vi "OptoSpike.vi"(8 "Threshold (mV)":dbl, 9 "Parameters for Optic stimulation":T1, 10 "Path of ABF file":path=path "C:/Users/KimYG/Documents/카카오톡 받은 파일/JJ_Ask for/PV_KO_Patch+other_10Hz_5ms.abf", 11 "OptoSpike Cluster IN":T2) -> (3 "OptoSpike Cluster OUT":T2)   [LabVIEW 2017]
uses:
  OptoSpike Cluster.ctl
  Parameters for Optic Stimulation.ctl
  <vilib>/addons/Wavelet Analysis/application.llb/WA Multiscale Peak Detection (Array).vi
  <vilib>/addons/_Advanced Signal Processing/NI_AdvSigProcWA.lvlib
panel:
  out "Epoch":sgl[][](graph)
  out "InterSpike Interval (sec)":string="1\t10\t100\n2\t11\t110\n3\t12\t120\n4\t13\t130\n5\t14\t140\n6\t15\t150\n7\t16\t160\n8\t17\t170\n9\t18\t180\n"
  out "Summary Table":string[][](table)
  out "Raster plot":cluster{"location":dbl[], i32[]}[](graph)
  out "File Paramters":T3
  out "Whole Trace":sgl[][](graph)
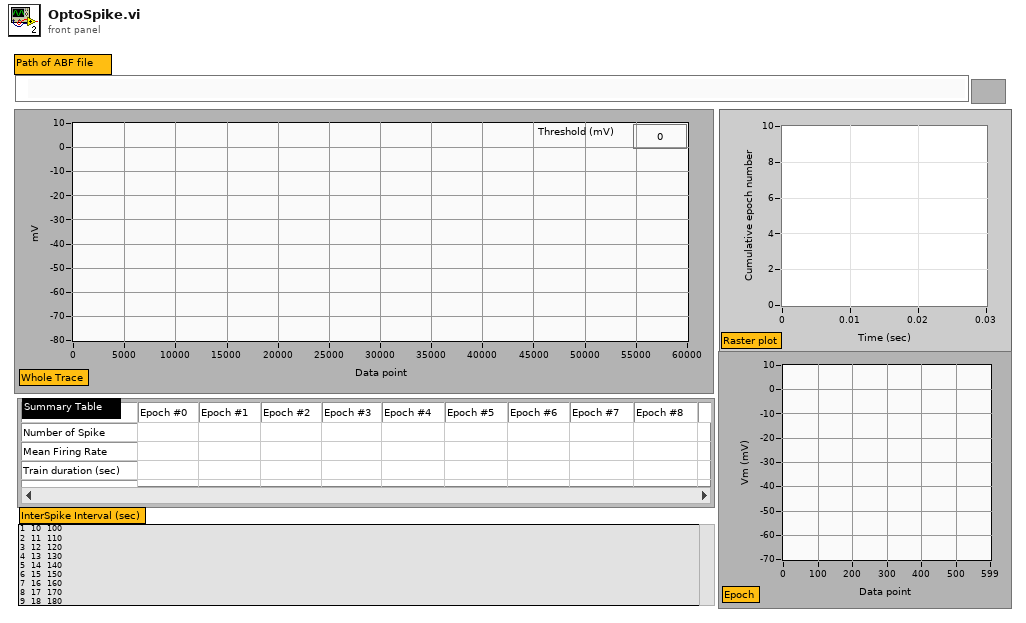
[diagram p1: front panel]
types:
  T1 = typedef "Parameters for Optic Stimulation.ctl" = cluster{"Begin (sec)":string, "Frequency (Hz)":string, "Epoch":string, "Time window (ms)":string}
  T2 = typedef "OptoSpike Cluster.ctl" = cluster{"File Paramters":cluster{"File Path":path, "Cell ID":string, "File Name":string, "Total Length":i32, "Trial Length (ms)":dbl, "Sweep Number":dbl, "Sampling rate":dbl}, "Raster Plot":cluster{"location":dbl[], "Sweep":i32[]}[], "Summary Table":string[][], "Pooled ISI":dbl[]}
  T3 = cluster{"File Path":path, "Cell ID":string, "File Name":string, "Total Length":i32, "Trial Length (ms)":dbl, "Sweep Number":dbl, "Sampling rate":dbl}
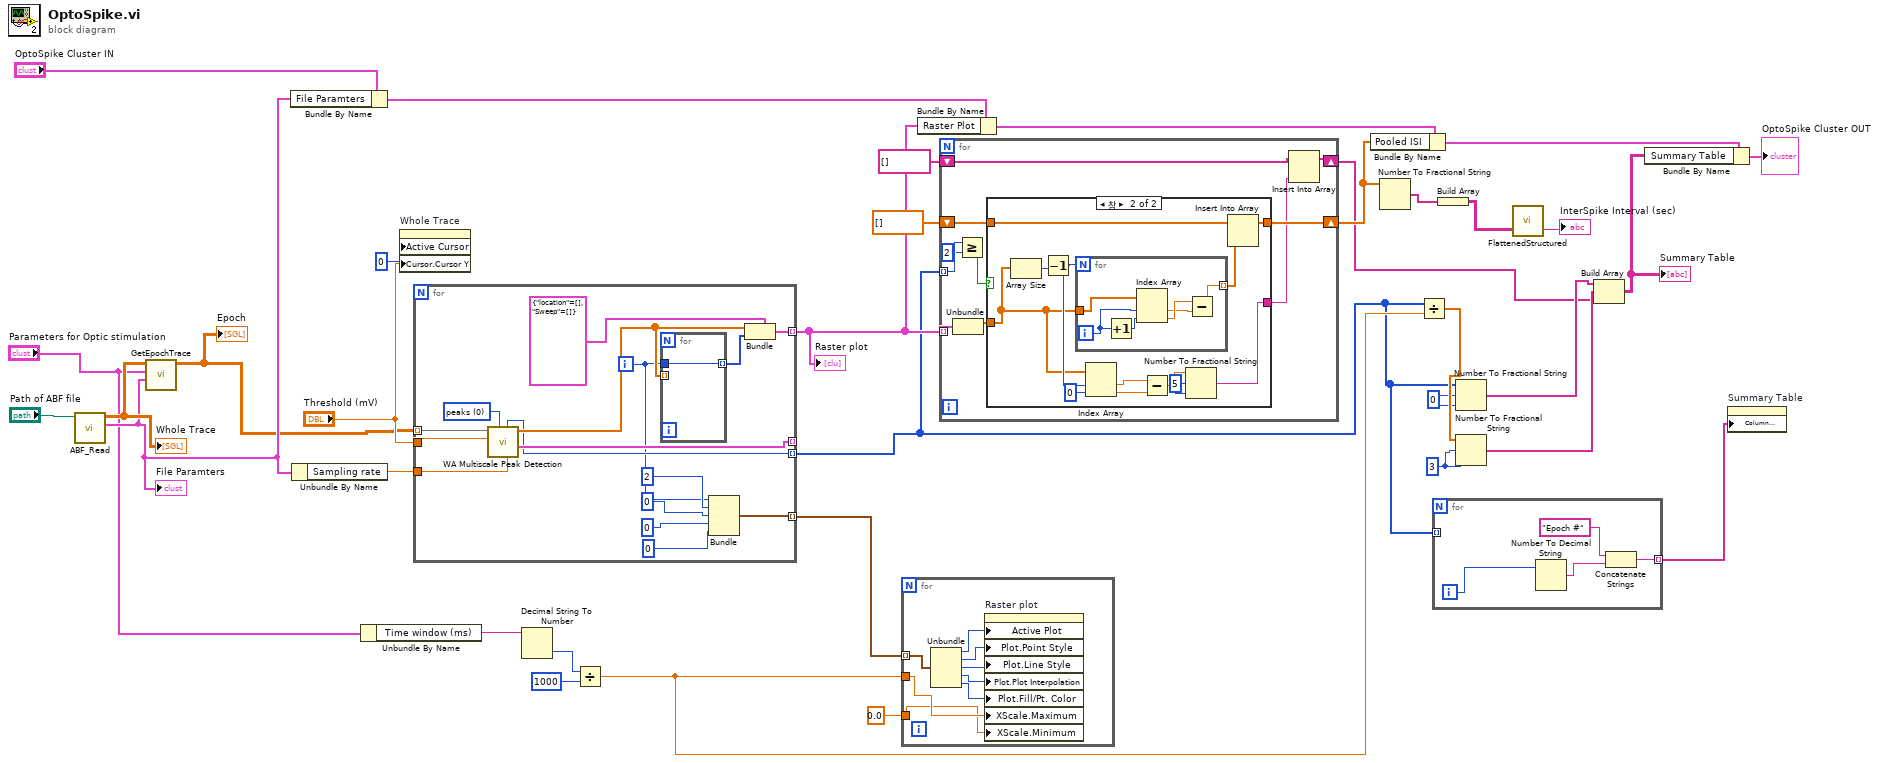
[diagram p0: block diagram]
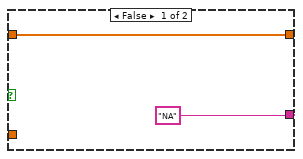
[diagram p2: hidden frame]
diagram:
  w7 = i16 3 ("폭(-)")
  w8 = i16 0 ("폭(-)")
  n1 = call "ABF_Read.vi"("Path of ABF file"="Path of ABF file") -> ("File Paramters"=w25:T3, "Whole Trace"=w26:sgl[][])  [unwired: 4 in, 1 out]
  "Whole Trace" <- w26
  "File Paramters" <- w25
  n2 = call "GetEpochTrace.vi"("File Paramters"=w25, "Parameters for Optic stimulation"="Parameters for Optic stimulation", "Whole Trace"=w26) -> ("Epoch"=w3:sgl[][])  [unwired: 4 in]
  "Epoch" <- w3
  n3 = Bundle By Name(cluster="OptoSpike Cluster IN", "File Paramters"=w25) -> (w32:T2)
  n4 = Unbundle By Name(w25) -> ("Sampling rate"=w20:dbl)
  n5 = Unbundle By Name("Parameters for Optic stimulation") -> ("Time window (ms)"=w22:string)
  n6 = property on="Whole Trace" class="WFGraph (엄격한)"("Active Cursor"=u32 0 ("활성 커서"), "Cursor.Cursor Y"="Threshold (mV)") -> ()  [unwired: 2 in, 2 out]
  n7 = for {
    tunnel: w3 -> [w51] mode=indexing
    tunnel: "Threshold (mV)" -> [w50]
    tunnel: [w48] -> _ mode=indexing
    tunnel: w20 -> [w47]
    tunnel: [w44] -> w27 mode=indexing
    tunnel: [w43] -> w5 mode=indexing
    tunnel: [w36] -> w24 mode=indexing
    i -> [w37]
    w49 = u16 0 items=["peaks", "valleys"] ("peaks/valleys")
    n8 = call-poly <vilib>:"WA Multiscale Peak Detection.vi"("sampling rate"=w47, "peaks/valleys"=w49, "threshold"=w50, "signal"=w51) -> ("peak plot"=w48:cluster{"Ramp Pattern":dbl[], "X":dbl[]}[], "location"=w46:dbl[], "number of peaks"=w43:i32)  [unwired: 3 in, 2 out]
    n9 = for {
      tunnel: w46 -> [_] mode=indexing
      tunnel: w37 -> [w52]
      tunnel: [w52] -> w45 mode=indexing
    }
    n10 = Bundle(w37, u8 2, u8 0, u8 0, u32 0) -> (w36:cluster{i32, u8, u8, u8, u32})  [unwired: 1 in]
    n11 = Bundle(cluster=cluster{"location":dbl[], "Sweep":i32[]} {"location"=[], "Sweep"=[]} ("클러스터"), "location"=w46, "Sweep"=w45) -> (w44:cluster{"location":dbl[], "Sweep":i32[]})
  }
  "Raster plot" <- w27
  n12 = Decimal String To Number(string=w22) -> (number=w21:i32)  [unwired: 2 in, 1 out]
  n13 = Divide(x=w21, y=1000) -> (x/y=w17:dbl)
  n14 = for {
    tunnel: w24 -> [w60] mode=indexing
    tunnel: w17 -> [w54]
    tunnel: 0.0 -> [w53]
    n15 = Unbundle(w60) -> (w59:i32, w58:u8, w57:u8, w56:u8, w55:u32)
    n16 = property on="Raster plot" class="XYGraph (엄격한)"("Active Plot"=w59, "Plot.Point Style"=w58, "Plot.Line Style"=w57, "Plot.Plot Interpolation"=w56, "Plot.Fill/Pt. Color"=w55, "XScale.Maximum"=w54, "XScale.Minimum"=w53) -> ()  [unwired: 2 in, 2 out]
  }
  n17 = Bundle By Name(cluster=w32, "Raster Plot"=w27) -> (w31:T2)
  n18 = for {
    tunnel: w27 -> [w70] mode=indexing
    shift-right: [w65] -> w15
    shift-left: dbl[] [] -> [w64]
    tunnel: w5 -> [w68] mode=indexing
    shift-right: [w62] -> w2
    shift-left: string[] [] -> [w61]
    n19 = Unbundle(w70) -> ("location"=w69:dbl[])  [unwired: 1 out]
    n20 = Greater Or Equal?(x=w68, y=2) -> (x >= y?=w66:bool)
    n21 = case shown="참" w66 {
      tunnel: w69 -> [_ w78]
      tunnel: w64 -> [w72 w81]
      tunnel: [w72 w82] -> w65
      tunnel: ["NA" w74] -> w63
      frame False {
      }
      frame True {
        w73 = i16 5 ("폭(-)")
        n22 = Array Size(array=w78) -> (size(s)=w84:i32)
        n23 = Decrement(x=w84) -> (x-1=w80:i32)
        n24 = for {
          N: w80 -> [_]
          tunnel: w78 -> [w90]
          tunnel: [w85] -> w83 mode=indexing
          i -> [w89]
          n25 = Increment(x=w89) -> (x+1=w88:i32)
          n26 = Index Array(array=w90, index #1=w89, index #2=w88) -> (element #1=w86:dbl, element #2=w87:dbl)
          n27 = Subtract(x=w87, y=w86) -> (x-y=w85:dbl)
        }
        n28 = Index Array(array=w78, index #1=w80, index #2=0 ("인덱스")) -> (element #1=w77:dbl, element #2=w76:dbl)
        n29 = Subtract(x=w77, y=w76) -> (x-y=w75:dbl)
        n30 = Number To Fractional String(number=w75, width (-)=w73, precision (6)=w73) -> (F-format string=w74:string)  [unwired: 1 in]
        n31 = Insert Into Array(array=w81, new element=w83) -> (w82:dbl[])  [unwired: 1 in]
      }
    }
    n32 = Insert Into Array(array=w61, new element=w63) -> (w62:string[])  [unwired: 1 in]
  }
  n33 = Bundle By Name(cluster=w31, "Pooled ISI"=w15) -> (w30:T2)
  n34 = Number To Fractional String(number=w15) -> (F-format string=w14:string[])  [unwired: 3 in]
  n35 = Divide(x=w5, y=w17) -> (x/y=w10:dbl[])
  n36 = for {
    tunnel: w5 -> [_] mode=indexing
    tunnel: [w91] -> w4 mode=indexing
    i -> [w94]
    n37 = Number To Decimal String(number=w94) -> (decimal integer string=w92:string)  [unwired: 1 in]
    n38 = Concatenate Strings("Epoch #", w92) -> (w91:string)
  }
  n39 = Build Array(w14) -> (w13:string[][])
  n40 = Number To Fractional String(number=w5, width (-)=w8, precision (6)=w8) -> (F-format string=w11:string[])  [unwired: 1 in]
  n41 = Number To Fractional String(number=w10, width (-)=w7, precision (6)=w7) -> (F-format string=w9:string[])  [unwired: 1 in]
  n42 = call <userlib>:"FlattenedStructured.vi"("Input (structured)"=w13) -> ("Output (flattened)"=→"InterSpike Interval (sec)":string)  [unwired: 1 in, 1 out]
  n43 = Build Array(w11, w9, w2) -> (w6:string[][])
  "Summary Table" <- w6
  n44 = Bundle By Name(cluster=w30, "Summary Table"=w6) -> (→"OptoSpike Cluster OUT":T2)
  n45 = property on="Summary Table" class="Tbl (엄격한)"("Column Headers[]"=w4) -> ()  [unwired: 2 in, 2 out]
